vi "WireWriteTagbusVIs.vi"(5 "terminals data":refnum<vi>[](array[refnum]), 7 "terminals indexes":refnum<vi>[](array[refnum]), 8 "error in":errorcluster, 9 "elements in cluster":i32, 10 "tag bus in in":refnum<vi>, 11 "VI in":refnum<vi>) -> (0 "error out":errorcluster, 2 "tag bus out":refnum<vi>, 3 "VI out":refnum<vi>)   [LabVIEW 2013, in "control module data interface generator.lvlib"]
uses:
  control module data interface generator.lvlib
  <vilib>/Utility/miscctls.llb/LVPointTypeDef.ctl
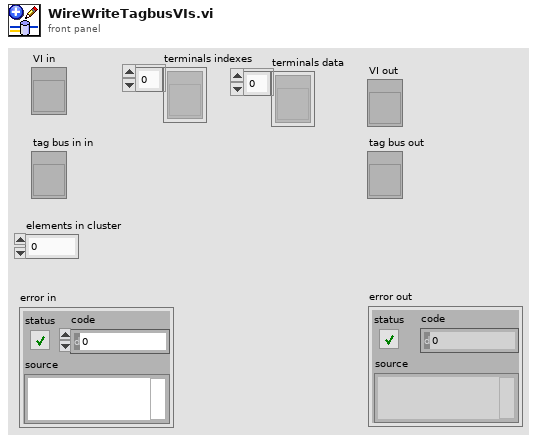
[diagram p1: front panel]
types:
  T1 = typedef "LVPointTypeDef.ctl" = cluster{"Horizontal":i16, "Vertical":i16}
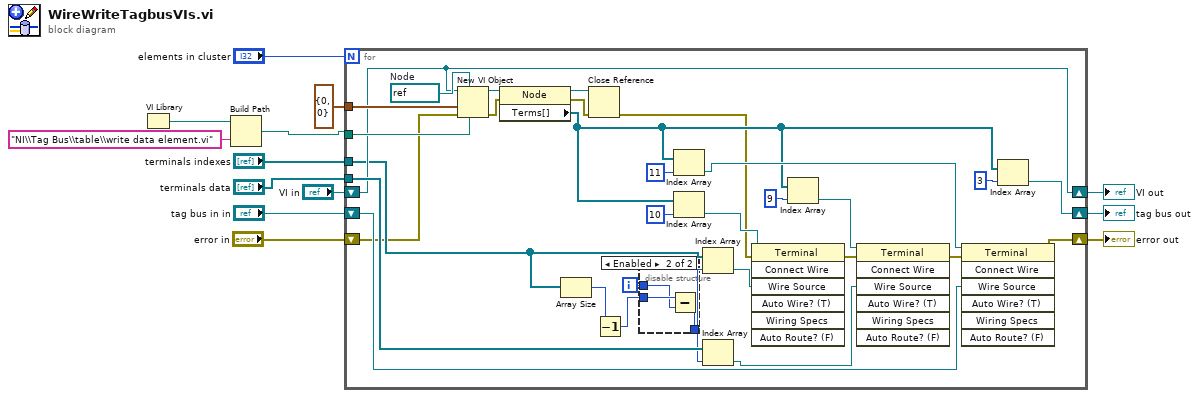
[diagram p0: block diagram]
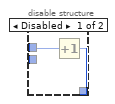
[diagram p2: hidden frame]
diagram:
  n1 = VI Library() -> (path=w2:path)
  n2 = Build Path(base path=w2, name or relative path="NI\\Tag Bus\\table\\write data element.vi") -> (appended path=w1:path)
  n3 = for {
    N: "elements in cluster" -> [_]
    tunnel: w1 -> [w44]
    tunnel: T1 {"Horizontal"=0, "Vertical"=0} ("location") -> [w43]
    tunnel: "terminals data" -> [w35]
    tunnel: "terminals indexes" -> [w19]
    shift-right: [w27] -> w11
    shift-left: "tag bus in in" -> [w30]
    shift-right: [w24] -> w10
    shift-left: "VI in" -> [w24]
    shift-right: [w20] -> w4
    shift-left: "error in" -> [w15]
    i -> [w26]
    w42 = refnum<vi> refnum  # Node
    n4 = New VI Object(vi object class=w42, owner refnum=w24, position/next to=w43, 6:w44, 8:w15) -> (object refnum=w37:refnum<vi>, 0:w16:errorcluster)  [unwired: 3 in]
    n5 = property on="Property Node" class="Node"(reference=w37, error in=w16) -> (reference out=w39:refnum<vi>, error out=w38:errorcluster, "Terms[]"=w23:refnum<vi>[])
    n6 = Array Size(array=w19) -> (size(s)=w18:i32)
    n7 = Close Reference(reference=w39, error in (no error)=w38) -> (error out=w14:errorcluster)
    n8 = Decrement(x=w18) -> (x-1=w17:i32)
    n9 = disable-structure shown="Enabled" {
      disable-tunnel: w26 -> [w46 w48]
      disable-tunnel: [w45 w47] -> w25
      disable-tunnel: w17 -> [_ w49]
      frame Disabled {
        n10 = Increment(x=w46) -> (x+1=w45:i32)
      }
      frame Enabled {
        n11 = Subtract(x=w49, y=w48) -> (x-y=w47:i32)
      }
    }
    n12 = Index Array(array=w23, index=11) -> (element=w29:refnum<vi>)
    n13 = Index Array(array=w23, index=10) -> (element=w33:refnum<vi>)
    n14 = Index Array(array=w19, index=w25) -> (element=w32:refnum<vi>)
    n15 = Index Array(array=w35, index=w25) -> (element=w34:refnum<vi>)
    n16 = invoke on="Invoke Node" class="Terminal" method="Connect Wire"(reference=w33, error in=w14, "Wire Source"=w32) -> (error out=w22:errorcluster)  [unwired: 4 in, 6 out]
    n17 = Index Array(array=w23, index=9) -> (element=w36:refnum<vi>)
    n18 = invoke on="Invoke Node" class="Terminal" method="Connect Wire"(reference=w36, error in=w22, "Wire Source"=w34) -> (error out=w21:errorcluster)  [unwired: 4 in, 6 out]
    n19 = invoke on="Invoke Node" class="Terminal" method="Connect Wire"(reference=w29, error in=w21, "Wire Source"=w30) -> (error out=w20:errorcluster)  [unwired: 4 in, 6 out]
    n20 = Index Array(array=w23, index=3) -> (element=w27:refnum<vi>)
  }
  "tag bus out" <- w11
  "VI out" <- w10
  "error out" <- w4
